vi "Speed Control 1-Before second motor.vi"(11 "queue in":refnum<queue>) -> ()   [LabVIEW 2014]
uses:
  controls/UI Data.ctl
  controls/EncoderController.ctl
  <vilib>/Platform/TimedLoop/XDataNode/timing_clust.ctl
  <vilib>/Platform/TimedLoop/XDataNode/nitl_modes.ctl
  <vilib>/Platform/TimedLoop/XDataNode/wakeup.ctl
  controls/Control StateSam.ctl
  controls/Control ConfigurationSam.ctl
  <vilib>/myRIO/Instrument Drivers/Onboard IO/PWM/typedefs/PWM Reference.ctl
  <vilib>/myRIO/Common/Instrument Driver Framework/Utilities/typedefs/myRIO Generic Hardware Reference.ctl
  <vilib>/myRIO/Common/Instrument Driver Framework/Utilities/typedefs/Hardware Version Enum.ctl
  <vilib>/myRIO/Common/Instrument Driver Framework/Utilities/typedefs/myRIO v1.0 Reference.ctl
  <vilib>/myRIO/Common/Instrument Driver Framework/Utilities/typedefs/Generic FPGA Reference.ctl
  <vilib>/myRIO/Common/Instrument Driver Framework/myRIO v1.0/PWM/typedefs/PWM Channels Enum.ctl
  <vilib>/myRIO/Instrument Drivers/Onboard IO/PWM/typedefs/PWM Configuration.ctl
  <vilib>/userdefined/High Color/nirio_resource_hc.ctl
  <vilib>/myRIO/Common/Instrument Driver Framework/Utilities/vis/Is FPGA Ref Available.vi
  <vilib>/myRIO/Common/Instrument Driver Framework/myRIO v1.0/PWM/vis/myRIO v1.1 Open PWM.vi
  <vilib>/myRIO/Instrument Drivers/Onboard IO/PWM/vis/Set Duty Cycle and Frequency.vi
  <vilib>/myRIO/Common/Instrument Driver Framework/Utilities/vis/Validate Channels.vi
  <vilib>/myRIO/Common/Instrument Driver Framework/myRIO v1.0/PWM/vis/myRIO v1.0 Reserve PWM.vi
  <vilib>/myRIO/Common/Instrument Driver Framework/myRIO v1.0/PWM/vis/myRIO v1.0 Build MUX Configuration PWM.vi
  <vilib>/myRIO/Common/Instrument Driver Framework/myRIO v1.0/Resource Manager/vis/myRIO v1.0 Reserve Channel List.vi
  <vilib>/myRIO/Common/Instrument Driver Framework/myRIO v1.0/Resource Manager/vis/myRIO v1.0 Create Configuration List.vi
  <vilib>/myRIO/Common/Instrument Driver Framework/myRIO v1.0/Resource Manager/vis/myRIO v1.0 Reserve Channel.vi
  <vilib>/myRIO/Common/Instrument Driver Framework/myRIO v1.0/Resource Manager/vis/myRIO v1.0 Unreserve Channel.vi
  <vilib>/myRIO/Common/Instrument Driver Framework/myRIO v1.0/Resource Manager/vis/myRIO v1.0 Build Mutex Name.vi
  <vilib>/Utility/VariantDataType/GetNumericInfo.vi
  <vilib>/Utility/error.llb/Error Cluster From Error Code.vi
  <vilib>/myRIO/Common/Instrument Driver Framework/myRIO v1.0/myRIO v1.1 Open.vi
  <vilib>/myRIO/Common/Instrument Driver Framework/Utilities/vis/IO Manager.vi
  <vilib>/myRIO/Common/Instrument Driver Framework/Utilities/vis/Configuration Manager.vi
  <vilib>/myRIO/Common/Instrument Driver Framework/myRIO v1.0/Resource Manager/vis/myRIO v1.0 Configure IO.vi
  <vilib>/myRIO/Common/Instrument Driver Framework/myRIO v1.0/myRIO v1.0 Close.vi
  <vilib>/myRIO/Common/Instrument Driver Framework/myRIO v1.0/PWM/vis/myRIO v1.0 Write PWM.vi
  <vilib>/Platform/TimedLoop/XDataNode/loadnilvce.vi
  <vilib>/addons/control/pid/pid.llb/PID (DBL).vi
  <vilib>/addons/control/pid/pid.llb/PID Percentage to EGU (DBL).vi
  <vilib>/myRIO/Express VI/Onboard IO/PWM/PWM Express VI.xnode
  <vilib>/myRIO/Instrument Drivers/Onboard IO/PWM/vis/myRIO PWM Open.xnode
  <vilib>/platform/TimedLoop/XDataNode/XDataNode.xnode
  <vilib>/addons/control/pid/NI_PID_pid.lvlib
  <vilib>/Platform/TimedLoop/XDataNode/XDNodeRunTimeDep.lvlib
  <vilib>/myRIO/Instrument Drivers/Onboard IO/PWM/PWM.lvlib
panel:
  out "Ch 4 Setpoint":dbl
  out "Motor1Output":dbl
  out "Velocity1 RPM":dbl
  # "0.8, 0. 0 is stable but theres a large offset\nsystem is slow to settle, increase Ti"
  # "Kp=2.04, Ti=0.15, Td=0.0375"
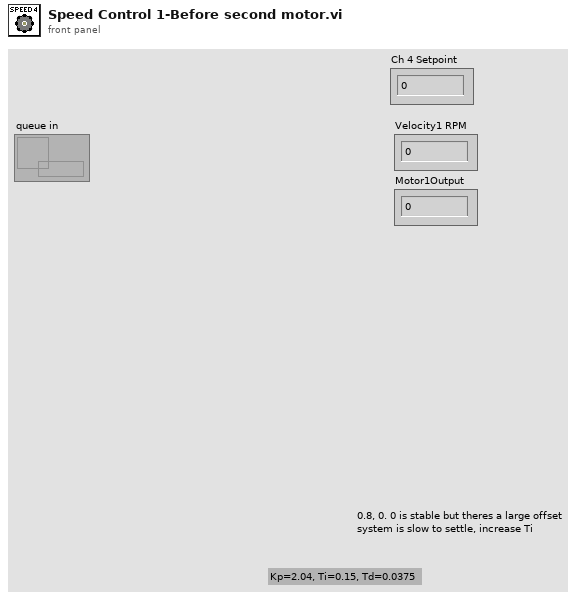
[diagram p1: front panel]
types:
  T1 = cluster{bool, "Tick Count(uSec)":u32, "Counter Value":i32, "x-y":i32}
  T2 = typedef "XDNodeRunTimeDep.lvlib/timing_clust.ctl" = cluster{"Expected End [f-1]":u64, "Actual End [f-1]":u64, "Finished Late? [f-1]":bool, "Expected End [i-1]":u64, "Actual End [i-1]":u64, "Finished Late? [i-1]":bool, "Expected Start [i]":u64, "Actual Start [i]":u64, "Expected Start [f]":u64, "Actual Start [f]":u64, "Source Name":string, "Structure Name":string, "Period":i64, "Deadline":i64, "Offset":i64, "Start":i64, "Priority":i32, "Timeout":i32, "Mode":T3, "Wakeup Reason":T4, "Error":errorcluster, "Source Type":string, "Secondary Source Type":string, "Global End Time":u64, "Global Start Time":u64, "Frame Duration":u64, "Iteration Duration":u64, "Assigned CPU":i32, "I/O Scan Engine Mode":u32}
  T3 = typedef "XDNodeRunTimeDep.lvlib/nitl_modes.ctl" = enum32{"No Change", "Process missed periods, maintain original phase", "Discard missed periods, maintain original phase", "Process missed periods, ignore original phase", "Discard missed periods, ignore original phase"}
  T4 = typedef "XDNodeRunTimeDep.lvlib/wakeup.ctl" = enum32{"Normal", "Aborted", "Asynchronous wakeup", "Timing source error", "Timed loop error", "Timeout"}
  T5 = typedef "Control StateSam.ctl" = enum16{"", "Control State (PID)", "Safe State"}
  T6 = typedef "Control ConfigurationSam.ctl" = cluster{"PID Gains":cluster{"proportional gain (Kc)":dbl, "integral gain (Kc*Ts/Ti)":dbl, "derivative gain (Kc*Td/Ts)":dbl}, "Output Range":cluster{"output high":dbl, "output low":dbl}}
  T7 = cluster{"proportional gain (Kc)":dbl, "integral gain (Kc*Ts/Ti)":dbl, "derivative gain (Kc*Td/Ts)":dbl}
  T8 = typedef "PWM.lvlib/PWM Reference.ctl" = cluster{"myRIO Reference":T9, "PWM Channels Enum":T13, "PWM Configuration":T14}
  T9 = typedef "myRIO Generic Hardware Reference.ctl" = cluster{"myRIO Model":T10, "myRIO Hardware Reference":T11}
  T10 = typedef "Hardware Version Enum.ctl" = enum16{"Unknown", "myRIO-1900", "myRIO-1950"}
  T11 = typedef "myRIO v1.0 Reference.ctl" = cluster{"Generic FPGA Reference":T12, "Allow multiple opens":bool}
  T12 = typedef "Generic FPGA Reference.ctl" = refnum<k20>
  T13 = typedef "PWM Channels Enum.ctl" = enum16{"Not Connected", "C/PWM0", "C/PWM1", "A/PWM0", "A/PWM1", "A/PWM2", "B/PWM0", "B/PWM1", "B/PWM2"}
  T14 = typedef "PWM.lvlib/PWM Configuration.ctl" = cluster{"Frequency":dbl, "Duty Cycle":dbl}
  T15 = typedef "nirio_resource_hc.ctl" = tag
  T16 = typedef "EncoderController.ctl" = cluster{"Sample time (uS)":u32, "Reset":bool}
  T17 = typedef "EncoderIndicator.ctl" = cluster{"Position":dbl, "Velocity RPM":dbl, "Velocity RPS":dbl}
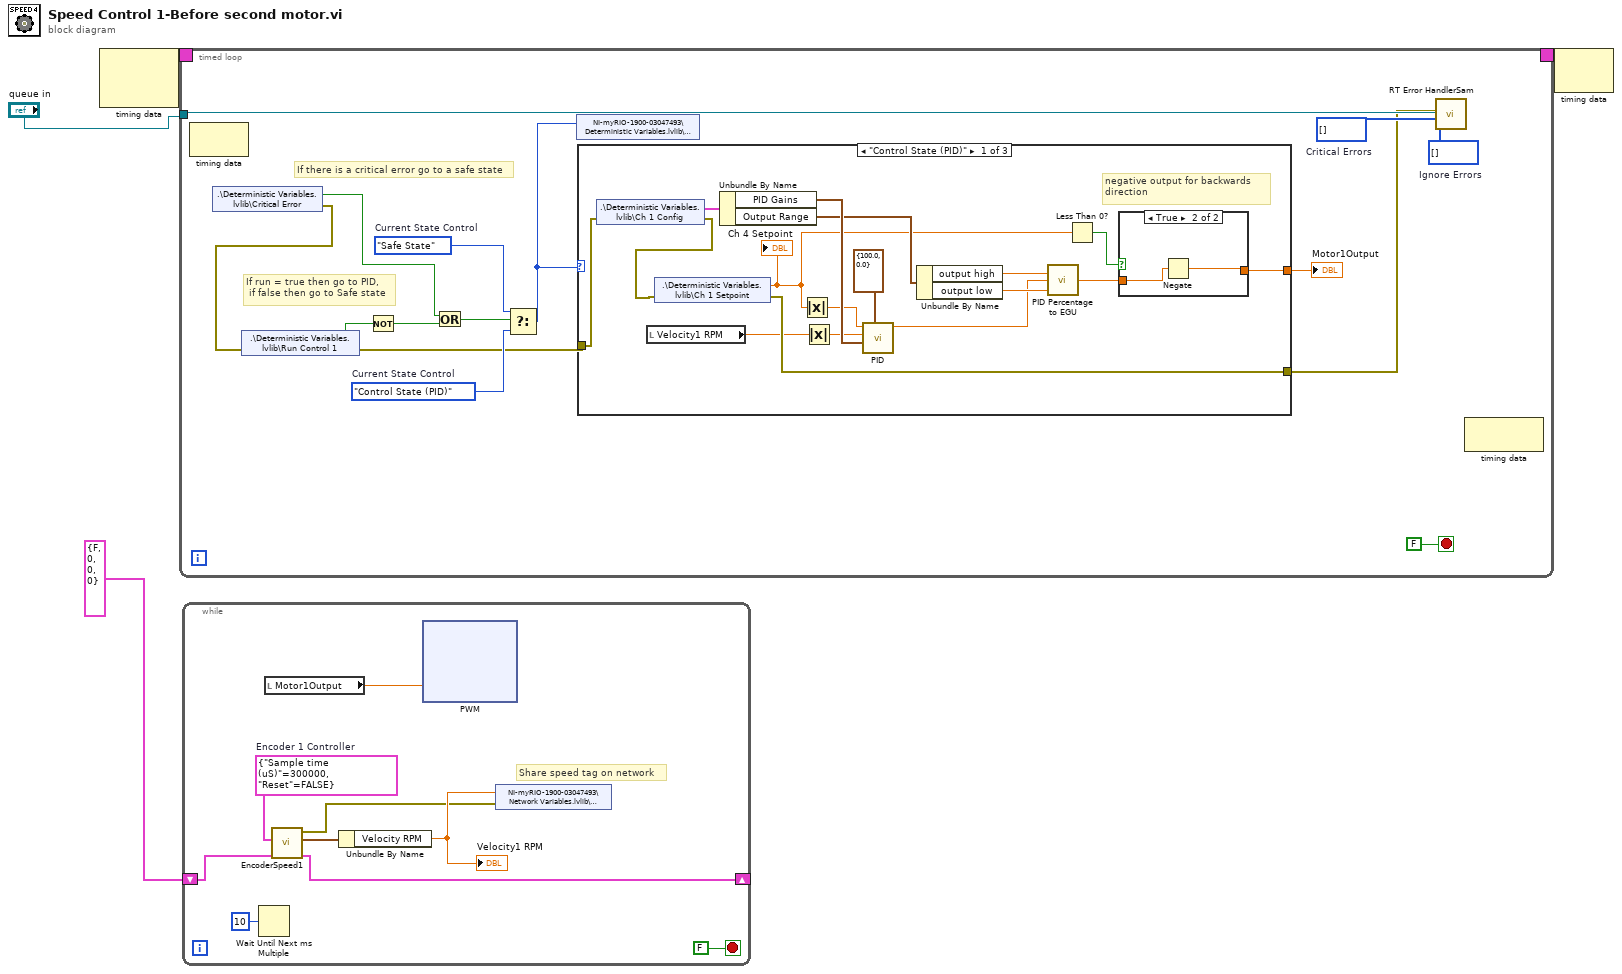
[diagram p0: block diagram]
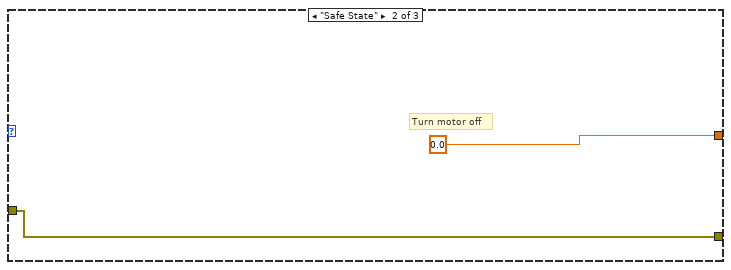
[diagram p3: hidden frame]
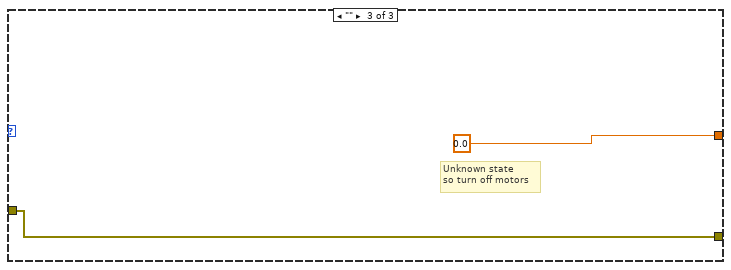
[diagram p4: hidden frame]
diagram:
  n1 = node-c288() -> (w4:T2)  [unwired: 2 in]
  n2 = timed-loop {
    timing: w4 -> [_]
    timing-out: [_] -> w3
    tunnel: "queue in" -> [w7]
    stop <- FALSE stop-if-true
    w8 = i32[] []  # Critical Errors
    w9 = i32[] []  # Ignore Errors
    w16 = Control_StateSam."Control State (PID)"  # Current State Control
    w17 = Control_StateSam."Safe State"  # Current State Control
    # "If there is a critical error go to a safe state"
    # "If run = true then go to PID,\n if false then go to Safe state"
    n3 = node-c288() -> ()  [unwired: 1 in, 1 out]
    n4 = shared-variable ".\\Deterministic Variables.lvlib\\Critical Error"() -> (w13:bool, error out=w11:errorcluster)  [unwired: 1 in]
    n5 = shared-variable ".\\Deterministic Variables.lvlib\\Run Control 1"(error in=w11) -> (w18:bool, error out=w10:errorcluster)
    n6 = Not(x=w18) -> (.not. x?=w14:bool)
    n7 = Or(x=w13, y=w14) -> (x .or. y?=w12:bool)
    n8 = Select(t=w17, s=w12, f=w16) -> (s? t:f=w15:T5)
    n9 = shared-variable "NI-myRIO-1900-03047493\\Deterministic Variables.lvlib\\Control State 1"(w15) -> ()  [unwired: 1 in, 1 out]
    n10 = case shown="\"Control State (PID)\"" w15 {
      tunnel: [w24 0.0 ("output (EGU)") 0.0 ("output (EGU)")] -> w6
      tunnel: w10 -> [w29 w40 w42]
      tunnel: [w27 w40 w42] -> w5
      frame "Control State (PID)" {
        # "negative output for backwards \ndirection"
        n11 = shared-variable ".\\Deterministic Variables.lvlib\\Ch 1 Config"(error in=w29) -> (w33:T6, error out=w28:errorcluster)
        n12 = local read "Velocity1 RPM"() -> (w21:dbl)
        n13 = shared-variable ".\\Deterministic Variables.lvlib\\Ch 1 Setpoint"(error in=w28) -> (w23:dbl, error out=w27:errorcluster)
        "Ch 4 Setpoint" <- w23
        n14 = Unbundle By Name(w33) -> ("PID Gains"=w34:T7, "Output Range"=w31:cluster{"output high":dbl, "output low":dbl})
        n15 = Absolute Value(x=w23) -> (abs(x)=w22:dbl)
        n16 = Absolute Value(x=w21) -> (abs(x)=w20:dbl)
        n17 = call-poly <vilib>:"PID.vi"("output range"=cluster{"output high":dbl, "output low":dbl} {"output high"=100.0, "output low"=0.0}, "PID gains"=w34, "process variable"=w20, "setpoint"=w22) -> ("output"=w32:dbl)  [unwired: 6 in, 1 out]
        n18 = Unbundle By Name(w31) -> ("output high"=w36:dbl, "output low"=w35:dbl)
        n19 = call-poly <vilib>:"PID Percentage to EGU.vi"("minimum (EGU)"=w35, "% span"=w32, "maximum (EGU)"=w36) -> ("output (EGU)"=w25:dbl)  [unwired: 1 in]
        n20 = Less Than 0?(x=w23) -> (x < 0?=w26:bool)
        n21 = case shown="True" w26 {
          tunnel: w25 -> [w37 w39]
          tunnel: [w37 w38] -> w24
          frame False {
          }
          frame True {
            n22 = Negate(x=w39) -> (-x=w38:dbl)
          }
        }
      }
      frame "Safe State" {
        # "Turn motor off"
      }
      frame "" {
        # "Unknown state\nso turn off motors"
      }
    }
    "Motor1Output" <- w6
    n23 = call "RT Error HandlerSam.vi"("Ignore Errors"=w9, "Critical Errors"=w8, "error to process"=w5, "queue in"=w7) -> ()  [unwired: 7 in, 1 out]
    n24 = node-c288() -> ()  [unwired: 1 in, 1 out]
  }
  n25 = while {
    shift-right: [w49] -> _
    shift-left: T1 {FALSE, "Tick Count(uSec)"=0, "Counter Value"=0, "x-y"=0} ("Cluster out") -> [w50]
    stop <- FALSE stop-if-true
    w54 = T16 {"Sample time (uS)"=300000, "Reset"=FALSE}  # Encoder 1 Controller
    # "Share speed tag on network"
    n26 = Wait Until Next ms Multiple(millisecond multiple=u32 10) -> ()  [unwired: 1 out]
    n27 = local read "Motor1Output"() -> (w46:dbl)
    n28 = call "EncoderSpeed1.vi"("Cluster in"=w50, "Encoder 1 Controller"=w54) -> ("Cluster out"=w49:T1, "Encoder 1 Indicator"=w53:T17, "error out"=w51:errorcluster)  [unwired: 7 in]
    n29 = Unbundle By Name(w53) -> ("Velocity RPM"=w52:dbl)
    "Velocity1 RPM" <- w52
    n30 = xnode "PWM"("Duty Cycle"=w46) -> ()  [unwired: 1 in, 1 out]
    n31 = shared-variable "NI-myRIO-1900-03047493\\Network Variables.lvlib\\SpeedMotor1"(w52, error in=w51) -> ()  [unwired: 1 out]
  }
  n32 = node-c288(w3) -> ()  [unwired: 1 out]
